vi "DataRefGet.vi"(8 "error in (no error)":errorcluster caption="错误输入（无错误）", 11 "MainPage 输入":refnum<class "MainPage.lvclass">) -> (0 "error out":errorcluster caption="错误输出", 1 "非法引用句柄？":bool, 2 "通讯接口记录":T1, 3 "MainPage 输出":refnum<class "MainPage.lvclass">, 4 "数据记录引用":refnum<data-value>)   [LabVIEW 2019, in "MainPage.lvlib" / "MainPage.lvclass"]
uses:
  MainPage.lvclass
  MainPage.lvclass/MainPage.ctl
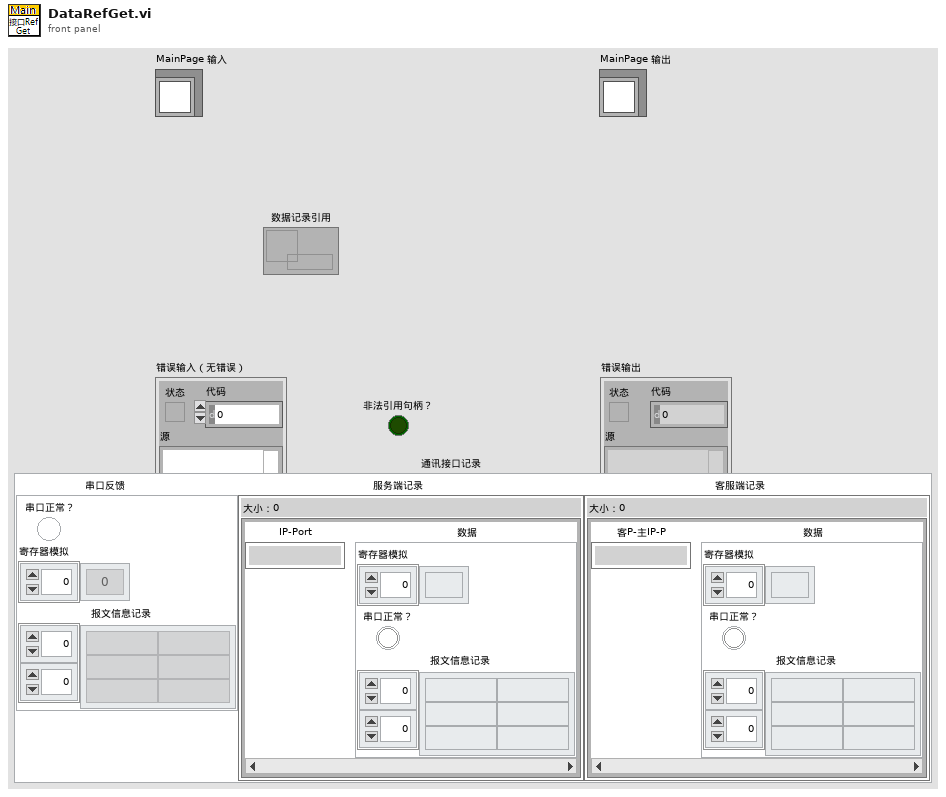
[diagram p1: front panel]
types:
  T1 = typedef "MainPage.lvlib/MainPage.lvclass/DataRef_通讯接口数据记录.ctl" = cluster{"串口反馈":cluster{"串口正常？":bool, "寄存器模拟":dbl[], "报文信息记录":string[][]}, "服务端记录":map{string, cluster{"寄存器模拟":dbl[], "串口正常？":bool, "报文信息记录":string[][]}}, "客服端记录":map{string, cluster{"寄存器模拟":dbl[], "串口正常？":bool, "报文信息记录":string[][]}}}
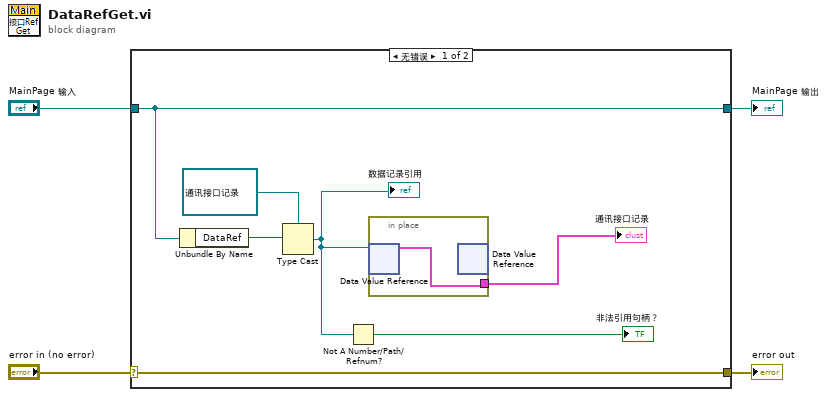
[diagram p0: block diagram]
diagram:
  n1 = case shown="无错误" "error in (no error)" {
    selector: "error in (no error)" -> [w11 w14]
    tunnel: [w11 w14] -> w3
    tunnel: [w10 w13] -> w1
    tunnel: "MainPage 输入" -> [w10 w13]
    frame No Error {
      n2 = Unbundle By Name(w10) -> ("DataRef"=w7:u32)
      n3 = Type Cast(type=refnum<data-value> refnum ("数据记录引用"), x=w7) -> (*(type *) &x=w8:refnum<data-value>)
      "数据记录引用" <- w8
      n4 = Not A Number/Path/Refnum?(number/path/refnum=w8) -> (NaN/Path/Refnum?=→"非法引用句柄？":bool)
      n5 = in-place {
        in-place-border: [w12] -> w5
        n6 = in-place-dvr #1(w8) -> (w12:T1)  [unwired: 1 out]
        n7 = in-place-dvr #1() -> ()  [unwired: 1 in, 2 out]
      }
      "通讯接口记录" <- w5
    }
    frame Error {
    }
  }
  "error out" <- w3
  "MainPage 输出" <- w1
